vi "Clusterwitharraysingle.vi"(1 "Cluster In":cluster{"Array In":sgl[], "Numeric Input":sgl} {"Numeric Input" format="%.2f"; "Array In" format="%.2f"}, 2 "Base":sgl format="%.2f") -> (0 "Cluster Out":cluster{"Array Out":sgl[], "Numeric Output":sgl} {"Numeric Output" format="%.2f"; "Array Out" format="%.2f"})   [LabVIEW 2012]
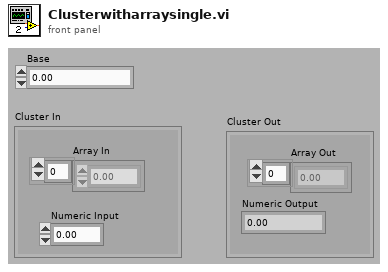
[diagram p1: front panel]
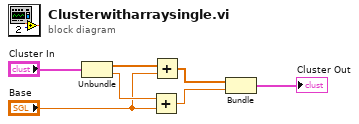
[diagram p0: block diagram]
diagram:
  n1 = Unbundle("Cluster In") -> ("Array In"=w7:sgl[], "Numeric Input"=w6:sgl)
  n2 = Add(x=w6, y="Base") -> (x+y=w4:sgl)
  n3 = Add(x=w7, y="Base") -> (x+y=w5:sgl[])
  n4 = Bundle(w5, w4) -> (→"Cluster Out":cluster{sgl[], sgl})  [unwired: 1 out]
